vi "parseValue.vi"(8 "error in (no error)":errorcluster, 10 "message":string, 11 "MonoClientCommunicator in":refnum<class "MonoClientCommunicator.lvclass">) -> (0 "error out":errorcluster, 1 "parameter":T1, 2 "value":variant, 3 "MonoClientCommunicator out":refnum<class "MonoClientCommunicator.lvclass">)   [LabVIEW 2016, in "MonoClientCommunicator.lvclass"]
uses:
  MonoClientCommunicator.lvclass
  Typedefs/publishers.ctl
  Typedefs/GratingType.ctl
  Typedefs/slitWidth.ctl
  Typedefs/DeviceStatus.ctl
  Typedefs/AckType.ctl
  Typedefs/wavelength.ctl
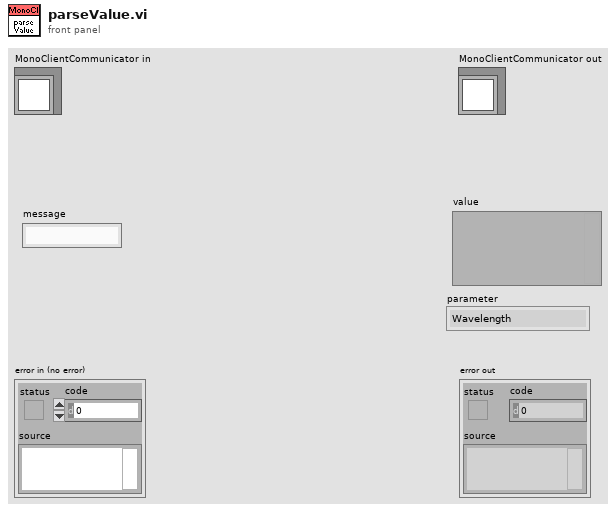
[diagram p1: front panel]
types:
  T1 = typedef "publishers.ctl" = enum16{"Wavelength", "Grating", "FrontEntranceSlitPosition", "FrontExitSlitPosition", "SoftwareStatus", "MonochromatorId", "Ack"}
  T2 = typedef "GratingType.ctl" = enum16{"Blue", "Red", "Mirror"}
  T3 = typedef "slitWidth.ctl" = dbl
  T4 = typedef "DeviceStatus.ctl" = enum16{"SettingUp", "Ready", "Offline", "Fault"}
  T5 = typedef "AckType.ctl" = enum16{"OK", "OutOfRange", "Unknown", "Busy", "Rejected"}
  T6 = typedef "wavelength.ctl" = dbl
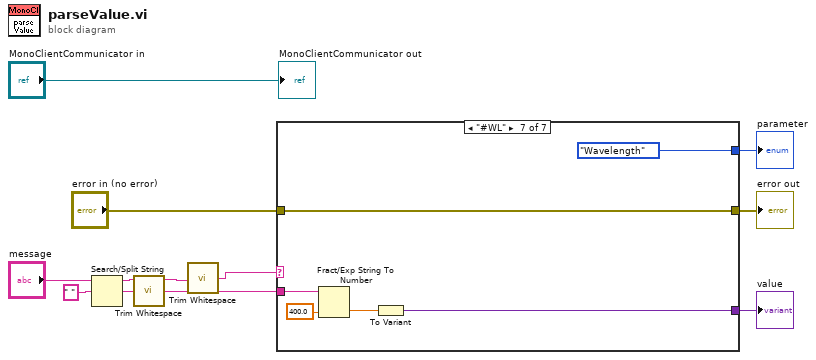
[diagram p0: block diagram]
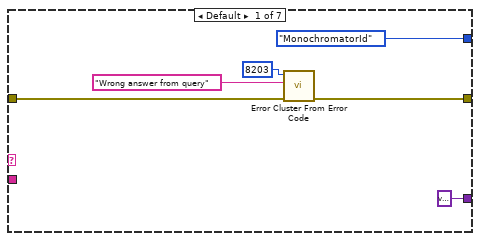
[diagram p2: hidden frame]
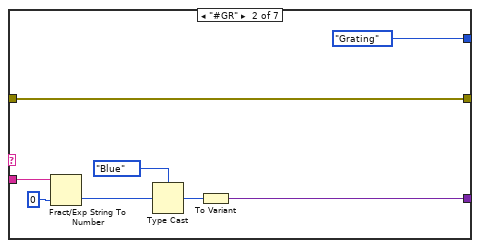
[diagram p3: hidden frame]
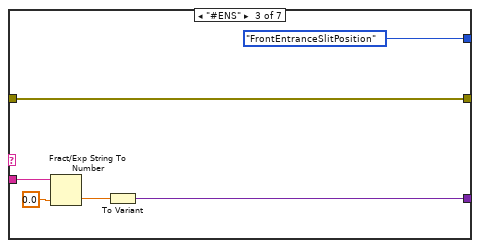
[diagram p4: hidden frame]
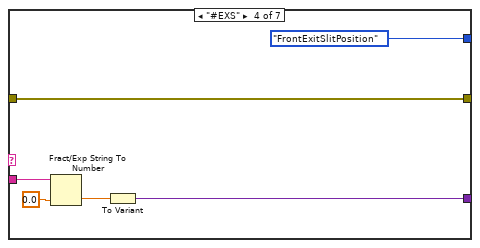
[diagram p5: hidden frame]
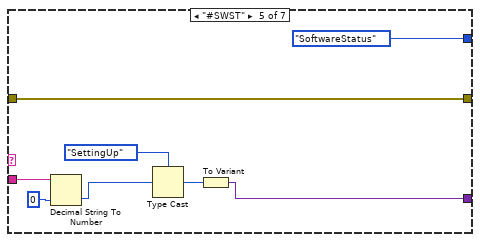
[diagram p6: hidden frame]
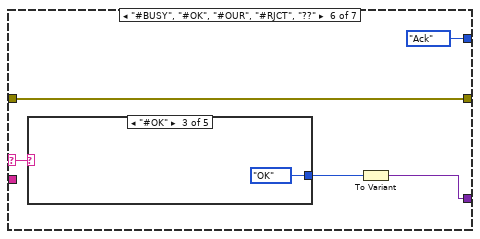
[diagram p7: hidden frame]
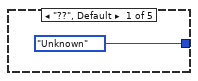
[diagram p8: hidden frame]
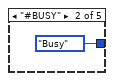
[diagram p9: hidden frame]
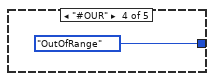
[diagram p10: hidden frame]
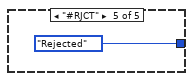
[diagram p11: hidden frame]
diagram:
  n1 = Search/Split String(string="message", search string/char (-)=" ") -> (substring before match=w2:string, match + rest of string=w8:string)  [unwired: 1 in, 1 out]
  n2 = call <vilib>:"Trim Whitespace.vi"("string"=w8) -> ("trimmed string"=w7:string)  [unwired: 1 in]
  n3 = call <vilib>:"Trim Whitespace.vi"("string"=w2) -> ("trimmed string"=w1:string)  [unwired: 1 in]
  n4 = case shown="\"#WL\"" w1 {
    selector: w1 -> [_ _ _ _ _ w47 _]
    tunnel: w7 -> [_ w24 w28 w34 w45 _ w61]
    tunnel: [variant ("Variant") w25 w30 w36 w41 w48 w58] -> w6
    tunnel: "error in (no error)" -> [w16 w18 w26 w32 w39 w50 w56]
    tunnel: [w15 w18 w26 w32 w39 w50 w56] -> w4
    tunnel: [publishers."MonochromatorId" ("publishers") publishers."Grating" ("publishers") publishers."FrontEntranceSlitPosition" ("publishers") publishers."FrontExitSlitPosition" ("publishers") publishers."SoftwareStatus" ("publishers") publishers."Ack" ("publishers") publishers."Wavelength" ("publishers")] -> w3
    frame Default {
      n5 = call <vilib>:"Error Cluster From Error Code.vi"("error in (no error)"=w16, "error message (\"\")"="Wrong answer from query" ("error message (\"\")"), "error code (0)"=8203) -> ("error out"=w15:errorcluster)  [unwired: 6 in]
    }
    frame "#GR" {
      n6 = Fract/Exp String To Number(string=w24, default (0 dbl)=u16 0) -> (number=w21:u16)  [unwired: 2 in, 1 out]
      n7 = Type Cast(type=GratingType."Blue" ("GratingType"), x=w21) -> (*(type *) &x=w22:T2)
      n8 = To Variant(anything=w22) -> (Variant=w25:variant)
    }
    frame "#ENS" {
      n9 = Fract/Exp String To Number(string=w28, default (0 dbl)=T3 0.0 ("position")) -> (number=w31:dbl)  [unwired: 2 in, 1 out]
      n10 = To Variant(anything=w31) -> (Variant=w30:variant)
    }
    frame "#EXS" {
      n11 = Fract/Exp String To Number(string=w34, default (0 dbl)=T3 0.0 ("position")) -> (number=w37:dbl)  [unwired: 2 in, 1 out]
      n12 = To Variant(anything=w37) -> (Variant=w36:variant)
    }
    frame "#SWST" {
      n13 = Decimal String To Number(string=w45, default (0L)=u16 0 ("default (0 I32)")) -> (number=w38:u16)  [unwired: 1 in, 1 out]
      n14 = Type Cast(type=DeviceStatus."SettingUp" ("DeviceStatus"), x=w38) -> (*(type *) &x=w42:T4)
      n15 = To Variant(anything=w42) -> (Variant=w41:variant)
    }
    frame "#BUSY", "#OK", "#OUR", "#RJCT", "??" {
      n16 = case shown="\"#OK\"" w47 {
        tunnel: [AckType."Unknown" ("Ack") AckType."Busy" ("Ack") AckType."OK" ("Ack") AckType."OutOfRange" ("Ack") AckType."Rejected" ("Ack")] -> w46
        frame "??", Default {
        }
        frame "#BUSY" {
        }
        frame "#OK" {
        }
        frame "#OUR" {
        }
        frame "#RJCT" {
        }
      }
      n17 = To Variant(anything=w46) -> (Variant=w48:variant)
    }
    frame "#WL" {
      n18 = Fract/Exp String To Number(string=w61, default (0 dbl)=T6 400.0 ("wavelength")) -> (number=w59:dbl)  [unwired: 2 in, 1 out]
      n19 = To Variant(anything=w59) -> (Variant=w58:variant)
    }
  }
  "error out" <- w4
  "value" <- w6
  "parameter" <- w3
  "MonoClientCommunicator out" <- "MonoClientCommunicator in"
